vi "Send.vi"   [LabVIEW 2025, in "ZeroMQ.lvlib" / "Socket.lvclass"]
uses:
  Socket.lvclass
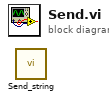
[diagram p0: block diagram]
diagram:
  n1 = call "Send_string.vi"() -> ()  [unwired: 10 in, 2 out]
